vi "Rohde & Schwarz VNA Read Status Bytes.vi"(7 "Rohde & Schwarz VNA":T1, 8 "error in (no error)":errorcluster, 10 "STB Only? (f: Read registers)":bool, 11 "VISA Resource Name":refnum<visa-resource-name>) -> (0 "error out":errorcluster, 2 "Event Status Register":bool[](array[boolean]), 3 "dup VISA Resource Name":refnum<visa-resource-name>, 4 "Status Byte":bool[](array[boolean]))   [LabVIEW 2011]
doc: "This VI for the HP8753B Network Analyzer reads the status byte and the two event status registers. The two status registers are read out as regular output and will therefore clear anything already in the output queue."
uses:
  TypeDefs/Rohde & Schwarz VNA Instrument Info.ctl
panel:
  # "read status byte only\nread status byte and status registers"
  # "Operation Complete\n\nRequest Control\n\nQuery Error\n\n\n\nExecution Error\n\nSyntax Error (GP-IB)\n\nUser Request\n\nPower On"
  # "Reverse GET\n\nForward GET\n\nEvent Status Register B\n\nCheck Error Queue\n\nMessage in Output Queue\n\nEvent Status Register\n\nRequest Service"
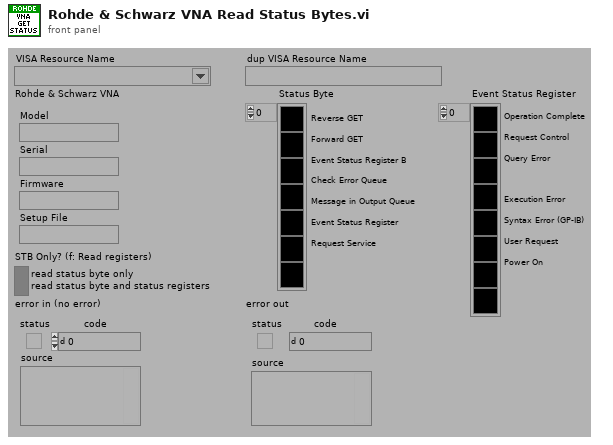
[diagram p1: front panel]
types:
  T1 = typedef "Rohde & Schwarz VNA Instrument Info.ctl" = cluster{"Model":string, "Serial":string, "Firmware":string, "Setup File":string}
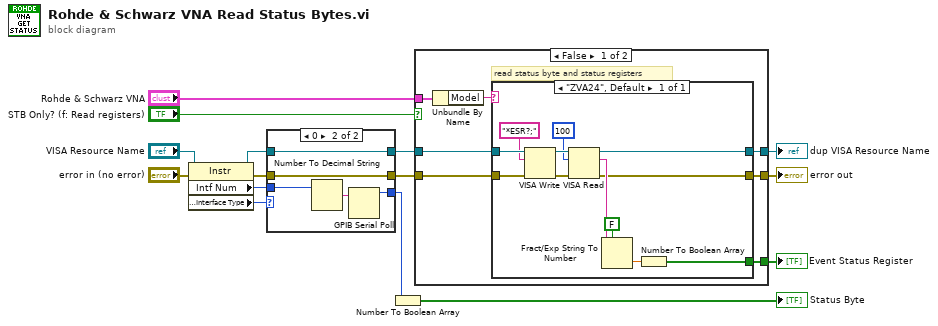
[diagram p0: block diagram]
diagram:
  n1 = property class="Instr"(reference="VISA Resource Name", error in="error in (no error)") -> (reference out=w5:refnum<visa-resource-name>, error out=w3:errorcluster, "Intf Num"=w1:u16, "Interface Information:Interface Type"=w2:u16)
  n2 = case shown="0" w2 {
    tunnel: [_ w22] -> w14
    tunnel: w5 -> [w17 w18]
    tunnel: [w17 w18] -> w13
    tunnel: [w16 w19] -> w10
    tunnel: w3 -> [w16 w19]
    tunnel: w1 -> [_ w20]
    frame Default {
    }
    frame 0 {
      n3 = Number To Decimal String(number=w20) -> (decimal integer string=w21:string)  [unwired: 1 out]
      n4 = GPIB Serial Poll(0:w21) -> (2:w22:i16)  [unwired: 1 in, 2 out]
    }
  }
  n5 = Number To Boolean Array(number=w14) -> (Boolean array=→"Status Byte":bool[])
  n6 = case shown="False" "STB Only? (f: Read registers)" {
    tunnel: w13 -> [w28 w43]
    tunnel: w10 -> [w29 w42]
    tunnel: [w27 w43] -> w12
    tunnel: [w26 w42] -> w11
    tunnel: "Rohde & Schwarz VNA" -> [w24 _]
    tunnel: [w25 _] -> w7
    frame False {
      # "read status byte and status registers"
      n7 = Unbundle By Name(w24) -> ("Model"=w23:string)
      n8 = case shown="\"ZVA24\", Default" w23 {
        tunnel: w29 -> [w41]
        tunnel: w28 -> [w40]
        tunnel: [w39] -> w25
        tunnel: [w30] -> w27
        tunnel: [w31] -> w26
        frame "ZVA24", Default {
          n9 = VISA Write(VISA resource name=w40, write buffer="*ESR?;", error in (no error)=w41) -> (VISA resource name out=w34:refnum<visa-resource-name>, error out=w37:errorcluster)  [unwired: 1 out]
          n10 = VISA Read(VISA resource name=w34, byte count=u32 100, error in (no error)=w37) -> (VISA resource name out=w30:refnum<visa-resource-name>, read buffer=w35:string, error out=w31:errorcluster)  [unwired: 1 out]
          n11 = Fract/Exp String To Number(use system decimal point (T)=FALSE, string=w35) -> (number=w36:dbl)  [unwired: 3 out]
          n12 = Number To Boolean Array(number=w36) -> (Boolean array=w39:bool[])
        }
      }
    }
    frame True {
      # "read status byte only"
    }
  }
  "dup VISA Resource Name" <- w12
  "error out" <- w11
  "Event Status Register" <- w7
